vi "He thong tuoi cay tu dong (2).vi"() -> ()   [LabVIEW 2025]
uses:
  <vilib>/Instr/_visa.llb/VISA Configure Serial Port (Instr).vi
panel:
  out "Hen gio":bool
  out "Tu dong":bool
  in  "Bang dieu khien":enum32{"Bat/Tat may bom", "Hen gio may bom"}(tab)
  in  "Bat may bom":bool
  in  "Tat may bom":bool
  out "LED Tin hieu":bool
  out "Thoi gian thuc 2":string
  in  "Thiet lap lai\nhen gio":bool caption="Reset"
  in  "Luon thiet lap lai":bool=TRUE caption="Auto Reset"
  in  "Tang 1 gio":bool
  in  "Giam 1 gio":bool
  out "Thoi gian bat dau hen gio:":string caption="Start Time Text"
  out "Thoi gian thuc":string caption="Present Text"
  out "Dem hen gio":dbl caption="Elapsed Time (s)"
  out "May gio sau bom":dbl
  out "%Do am":dbl(slide) scale=0.0..10.0
  out "Do thi":dbl(graph)
  in  "stop":bool
  in  "Cong ket noi":refnum<visa-resource-name>
  # "Che do ma mach dang su dung"
  # "Muon reset ngay thi bat autoreset truoc"
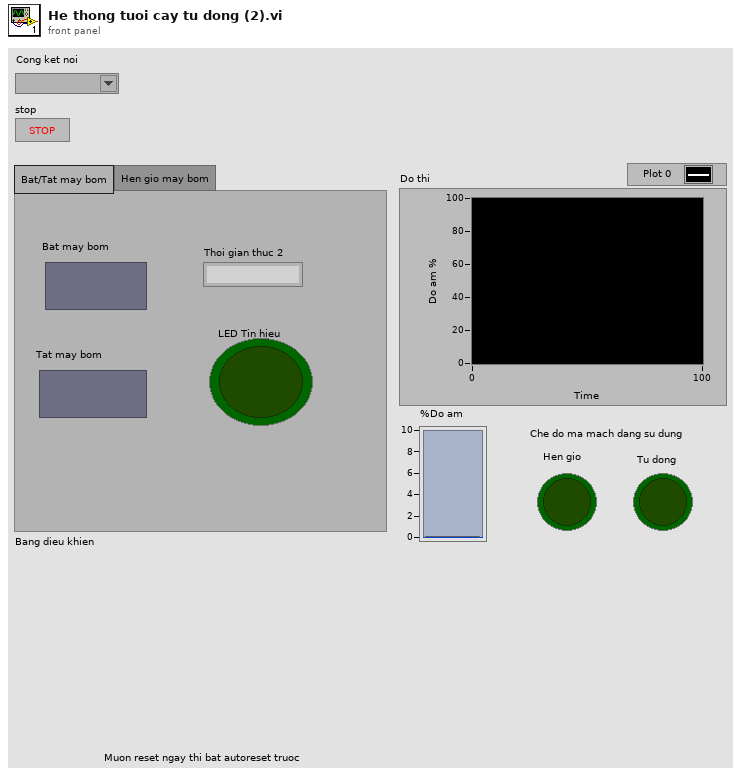
[diagram p1: front panel]
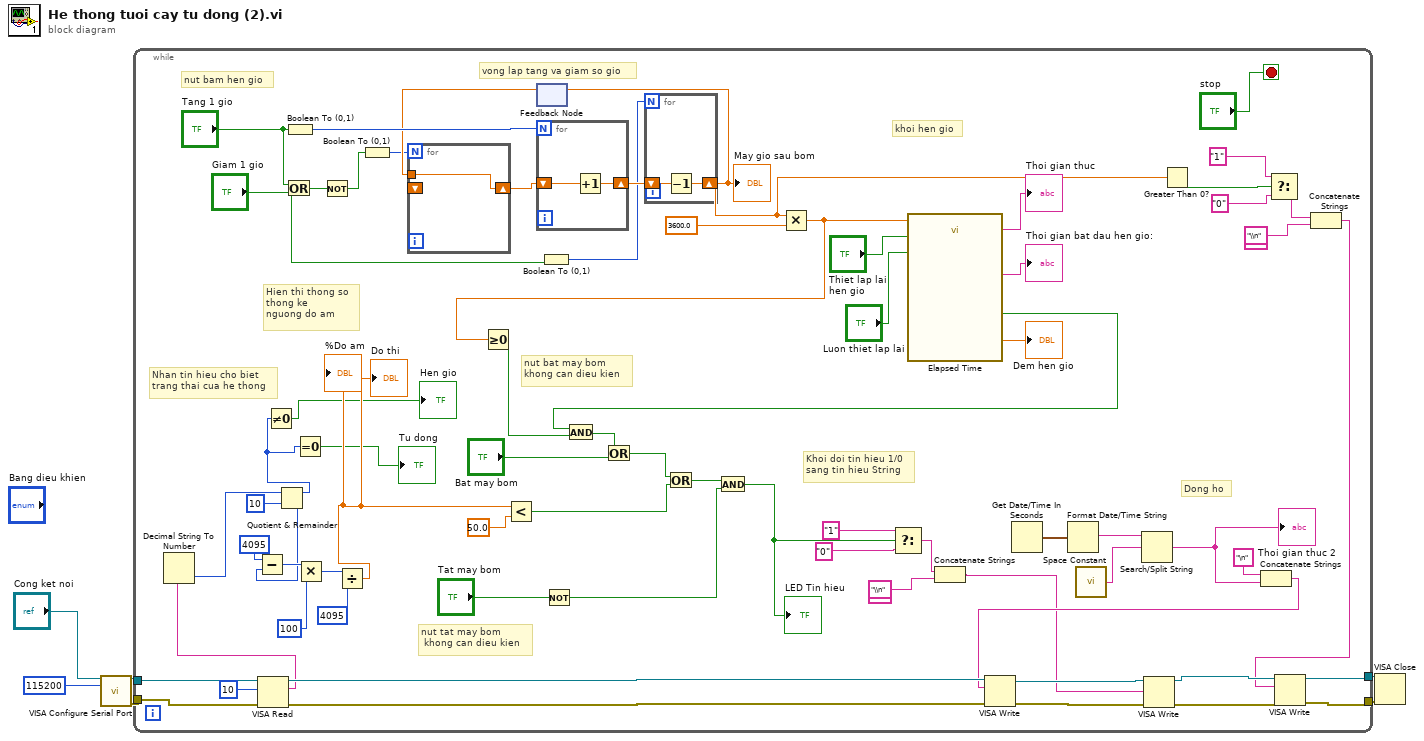
[diagram p0: block diagram]
diagram:
  n1 = call-poly "VISA Configure Serial Port"("VISA resource name"="Cong ket noi", "baud rate (9600)"=u32 115200) -> ("VISA resource name out"=w4:refnum<visa-resource-name>, "error out"=w3:errorcluster)  [unwired: 12 in]
  n2 = while {
    tunnel: w4 -> [w74]
    tunnel: w3 -> [w73]
    tunnel: [w16] -> w2
    tunnel: [w15] -> w1
    stop <- "stop" stop-if-true
    (unwired) "\\n" ("string")
    (unwired) "\\n" ("string")
    # "Nhan tin hieu cho biet \ntrang thai cua he thong"
    # "vong lap tang va giam so gio"
    # "khoi hen gio"
    # "Khoi doi tin hieu 1/0\nsang tin hieu String"
    # "Dong ho"
    # "nut tat may bom\n khong can dieu kien"
    # "nut bat may bom \nkhong can dieu kien"
    # "Hien thi thong so\nthong ke\nnguong do am"
    # "nut bam hen gio"
    n3 = VISA Read(VISA resource name=w74, byte count=u32 10, error in (no error)=w73) -> (VISA resource name out=w67:refnum<visa-resource-name>, read buffer=w66:string, error out=w40:errorcluster)  [unwired: 1 out]
    n4 = Decimal String To Number(string=w66) -> (number=w24:i32)  [unwired: 2 in, 1 out]
    n5 = Quotient & Remainder(x=w24, y=10) -> (x-y*floor(x/y)=w20:i32, floor(x/y)=w22:i32)
    n6 = Subtract(x=4095, y=w22) -> (x-y=w29:i32)
    n7 = Not Equal To 0?(x=w20) -> (x != 0?=→"Hen gio":bool)
    n8 = Or(x="Tang 1 gio", y="Giam 1 gio") -> (x .or. y?=w54:bool)
    n9 = Boolean To (0,1)(Boolean="Tang 1 gio") -> (0, 1=w58:i16)
    n10 = Equal To 0?(x=w20) -> (x = 0?=→"Tu dong":bool)
    n11 = Multiply(x=w29, y=100) -> (x*y=w27:i32)
    n12 = Not(x=w54) -> (.not. x?=w59:bool)
    n13 = Divide(x=w27, y=4095) -> (x/y=w25:dbl)
    "Do thi" <- w25
    "%Do am" <- w25
    n14 = Boolean To (0,1)(Boolean=w59) -> (0, 1=w51:i16)
    n15 = Less?(x=w25, y=50.0) -> (x < y?=w60:bool)
    n16 = feedback #1() -> (w57:dbl)  [unwired: 1 in]
    n17 = for {
      N: w51 -> [_]
      shift-right: [w81] -> w56
      shift-left: _ -> [_]
      tunnel: w57 -> [w81]
    }
    n18 = for {
      N: w58 -> [_]
      shift-right: [w80] -> w55
      shift-left: w56 -> [w79]
      n19 = Increment(x=w79) -> (x+1=w80:dbl)
    }
    n20 = Boolean To (0,1)(Boolean="Giam 1 gio") -> (0, 1=w52:i16)
    n21 = Not(x="Tat may bom") -> (.not. x?=w64:bool)
    n22 = for {
      N: w52 -> [_]
      shift-right: [w78] -> w18
      shift-left: w55 -> [w77]
      n23 = Decrement(x=w77) -> (x-1=w78:dbl)
    }
    "May gio sau bom" <- w18
    n24 = feedback-in #1(w18) -> ()
    n25 = Multiply(x=w18, y=3600.0) -> (x*y=w38:dbl)
    n26 = Greater Or Equal To 0?(x=w38) -> (x >= 0?=w37:bool)
    n27 = call "Elapsed Time"("Time Target (s)"=w38, "Reset"="Thiet lap lai\nhen gio", "Auto Reset"="Luon thiet lap lai") -> ("Start Time Text"=→"Thoi gian bat dau hen gio:":string, "Present Text"=→"Thoi gian thuc":string, "Elapsed Time (s)"=→"Dem hen gio":dbl, "Time has Elapsed"=w39:bool)  [unwired: 9 in, 4 out]
    n28 = And(x=w39, y=w37) -> (x .and. y?=w36:bool)
    n29 = Or(x=w36, y="Bat may bom") -> (x .or. y?=w43:bool)
    n30 = Or(x=w43, y=w60) -> (x .or. y?=w71:bool)
    n31 = And(x=w71, y=w64) -> (x .and. y?=w68:bool)
    "LED Tin hieu" <- w68
    n32 = Select(t="1", s=w68, f="0") -> (s? t:f=w11:string)
    n33 = Concatenate Strings(w11, "\\n" ("string")) -> (w31:string)
    n34 = Get Date/Time In Seconds() -> (seconds since 1Jan1904=w63:timestamp)
    n35 = Format Date/Time String(seconds (now)=w63) -> (date/time string=w62:string)  [unwired: 2 in]
    n36 = call <vilib>:"Space Constant.vi"() -> ("String"=w61:string)
    n37 = Search/Split String(string=w62, search string/char (-)=w61) -> (match + rest of string=w34:string)  [unwired: 1 in, 2 out]
    "Thoi gian thuc 2" <- w34
    n38 = Greater Than 0?(x=w18) -> (x > 0?=w12:bool)
    n39 = Concatenate Strings("\n" ("string"), w34) -> (w32:string)
    n40 = VISA Write(VISA resource name=w67, write buffer=w32, error in (no error)=w40) -> (VISA resource name out=w41:refnum<visa-resource-name>)  [unwired: 2 out]
    n41 = VISA Write(VISA resource name=w41, write buffer=w31, error in (no error)=w40) -> (VISA resource name out=w17:refnum<visa-resource-name>, error out=w14:errorcluster)  [unwired: 1 out]
    n42 = Select(t="1", s=w12, f="0") -> (s? t:f=w8:string)
    n43 = Concatenate Strings(w8, "\\n" ("string")) -> (w7:string)
    n44 = VISA Write(VISA resource name=w17, write buffer=w7, error in (no error)=w14) -> (VISA resource name out=w16:refnum<visa-resource-name>, error out=w15:errorcluster)  [unwired: 1 out]
  }
  n45 = VISA Close(VISA resource name=w2, error in (no error)=w1) -> ()  [unwired: 1 out]
